vi "Camera Configuration Settings.vi"() -> ()   [LabVIEW 2019]
uses:
  <vilib>/vision/driver/IMAQdx.llb/IMAQdx Attribute Type.ctl
  <vilib>/userDefined/High Color/IMAQdx.ctl
  <vilib>/vision/driver/IMAQdx.llb/IMAQdx Buffer Number Mode.ctl
  <vilib>/FPGAPlugInAG/myRIO-1900/niLvFpga_Open_myRIO-1900.vi
  <vilib>/rvi/interface/common/dynamic/niFpgaDynamicAddResources.vi
  <vilib>/rvi/interface/nirviOpenFPGA/nirviOpenFPGA.xnode
  Collin's Project/FPGA Bitfiles/MRmecanum_FPGATarget_FPGAMainModified_TerasRobot_LKSN2021.lvbitx
  <vilib>/vision/driver/NI_Vision_Acquisition_Software.lvlib
  <resource>/objmgr/imaqdx.rc
panel:
  out "Image":T1(plugin-control)
  in  "ValueI64 2":i64
  out "error out 2":errorcluster
  out "error out":errorcluster
  in  "Exposure":u16(slide)=3750 scale=1000.0..6500.0
  in  "stop":bool
  out "Attribute Information Array":T3(array[cluster])
  in  "error in":errorcluster
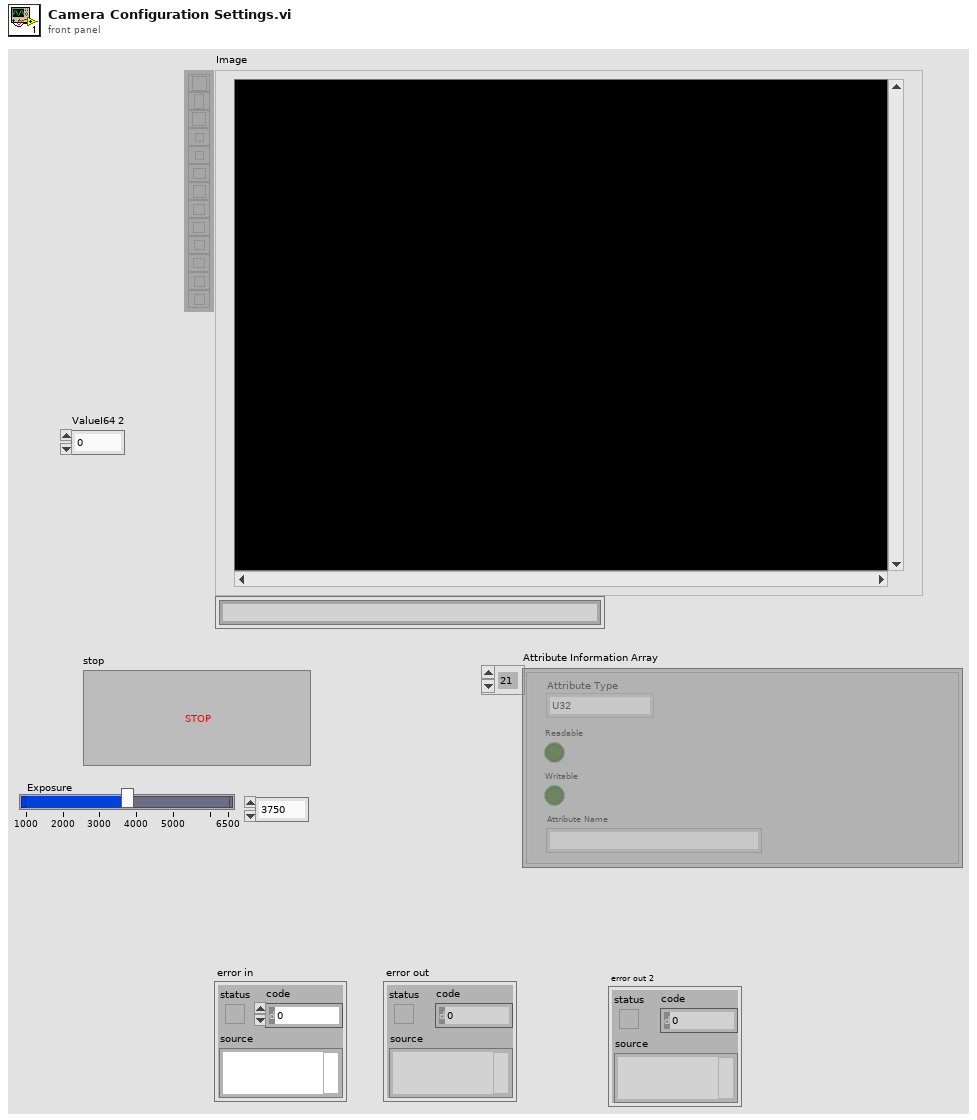
[diagram p1: front panel]
types:
  T1 = typedef "IMAQ Image.ctl" = refnum<image>
  T2 = typedef "NI_Vision_Acquisition_Software.lvlib/IMAQdx Attribute Type.ctl" = enum32{"U32", "I64", "DBL", "String", "Enum", "Bool", "Command"}
  T3 = cluster{"Attribute Type":T2, "Readable":bool, "Writable":bool, "Attribute Name":string}[]
  T4 = typedef "IMAQdx.ctl" = refnum<k21>
  T5 = typedef "NI_Vision_Acquisition_Software.lvlib/IMAQdx Buffer Number Mode.ctl" = enum32{"Next", "Last", "Buffer Number", "Every", "Last New"}
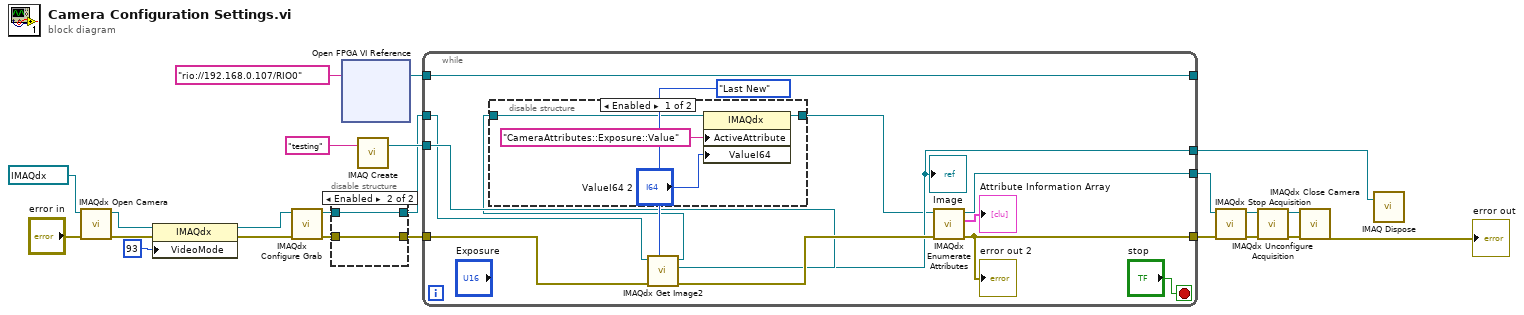
[diagram p0: block diagram]
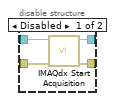
[diagram p2: hidden frame]
diagram:
  n1 = call <vilib>:"IMAQdx Open Camera.vi"("error in"="error in", "Session In"=T4 "cam1") -> ("error out"=w18:errorcluster, "Session Out"=w23:T4)  [unwired: 8 in]
  n2 = property class="IMAQdx"(reference=w23, error in=w18, "VideoMode"=u32 93) -> (reference out=w20:T4, error out=w17:errorcluster)
  n3 = call <vilib>:"IMAQdx Configure Grab.vi"("error in"=w17, "Session In"=w20) -> ("error out"=w15:errorcluster, "Session Out"=w16:T4)  [unwired: 8 in]
  n4 = disable-structure shown="Enabled" {
    disable-tunnel: w16 -> [w27 w29]
    disable-tunnel: w15 -> [w26 w28]
    disable-tunnel: [w25 w28] -> w10
    disable-tunnel: [w24 w29] -> w2
    frame Disabled {
      n5 = call <vilib>:"IMAQdx Start Acquisition.vi"("error in"=w26, "Session In"=w27) -> ("error out"=w25:errorcluster, "Session Out"=w24:T4)  [unwired: 8 in]
    }
    frame Enabled {
    }
  }
  n6 = xnode "Open FPGA VI Reference"("resource name"=tag "rio://192.168.0.107/RIO0") -> ("FPGA VI Reference Out"=w11:refnum<k20>)  [unwired: 1 in, 1 out]
  n7 = call "IMAQ Create"("Image Name"="testing") -> ("New Image"=w13:T1)  [unwired: 4 in, 1 out]
  n8 = while {
    tunnel: w13 -> [w34]
    tunnel: [w40] -> w8
    tunnel: w11 -> [w38]
    tunnel: [w38] -> _
    tunnel: w10 -> [w37]
    tunnel: [w35] -> w3
    tunnel: w2 -> [w31]
    tunnel: [w33] -> w1
    stop <- "stop" stop-if-true
    n9 = call <vilib>:"IMAQdx Get Image2.vi"("Buffer Number Mode (Next)"=IMAQdx_Buffer_Number_Mode."Last New", "error in"=w37, "Image In"=w34, "Session In"=w31) -> ("error out"=w36:errorcluster, "Image Out"=w33:T1, "Session Out"=w32:T4)  [unwired: 4 in, 1 out]
    "Image" <- w33
    n10 = disable-structure shown="Enabled" {
      disable-tunnel: w32 -> [w46 w47]
      disable-tunnel: [w44 w47] -> w30
      frame Enabled {
        n11 = property class="IMAQdx"(reference=w46, "ActiveAttribute"="CameraAttributes::Exposure::Value", "ValueI64"="ValueI64 2") -> (reference out=w44:T4)  [unwired: 1 in, 1 out]
      }
      frame Disabled {
      }
    }
    n12 = call <vilib>:"IMAQdx Enumerate Attributes.vi"("error in"=w36, "Session In"=w30) -> ("error out"=w35:errorcluster, "Attribute Information Array"=→"Attribute Information Array":T3, "Session Out"=w40:T4)  [unwired: 7 in]
    "error out 2" <- w35
  }
  n13 = call <vilib>:"IMAQdx Stop Acquisition.vi"("error in"=w3, "Session In"=w8) -> ("error out"=w4:errorcluster, "Session Out"=w7:T4)  [unwired: 8 in]
  n14 = call <vilib>:"IMAQdx Unconfigure Acquisition.vi"("error in"=w4, "Session In"=w7) -> ("error out"=w5:errorcluster, "Session Out"=w6:T4)  [unwired: 8 in]
  n15 = call <vilib>:"IMAQdx Close Camera.vi"("error in"=w5, "Session In"=w6) -> ("error out"=→"error out":errorcluster)  [unwired: 9 in]
  n16 = call "IMAQ Dispose"("Image"=w1) -> ()  [unwired: 5 in, 1 out]
